vi "Read Map Attributes.vi"(8 "error in":errorcluster, 11 "Tree Map In (empty)":T3) -> (0 "error out":errorcluster, 1 "Modules Types Out":T1[](array[typedef]), 2 "Library References":refnum<vi>[](array[refnum]), 3 "References":T2, 4 "Dependencies?":bool[](array[boolean]), 6 "Descriptions":string[](array[string]))   [LabVIEW 2019, in "Panther Dashboard.lvlib"]
uses:
  Panther Dashboard.lvlib
  <vilib>/National Instruments/Tree Map/Tree Map Data.ctl
  Project References--cluster.ctl
  Module type--enum.ctl
  Map Attribute--enum.ctl
  Panther Dashboard--global.vi
  <vilib>/National Instruments/Tree Map/Tree Map.lvlib
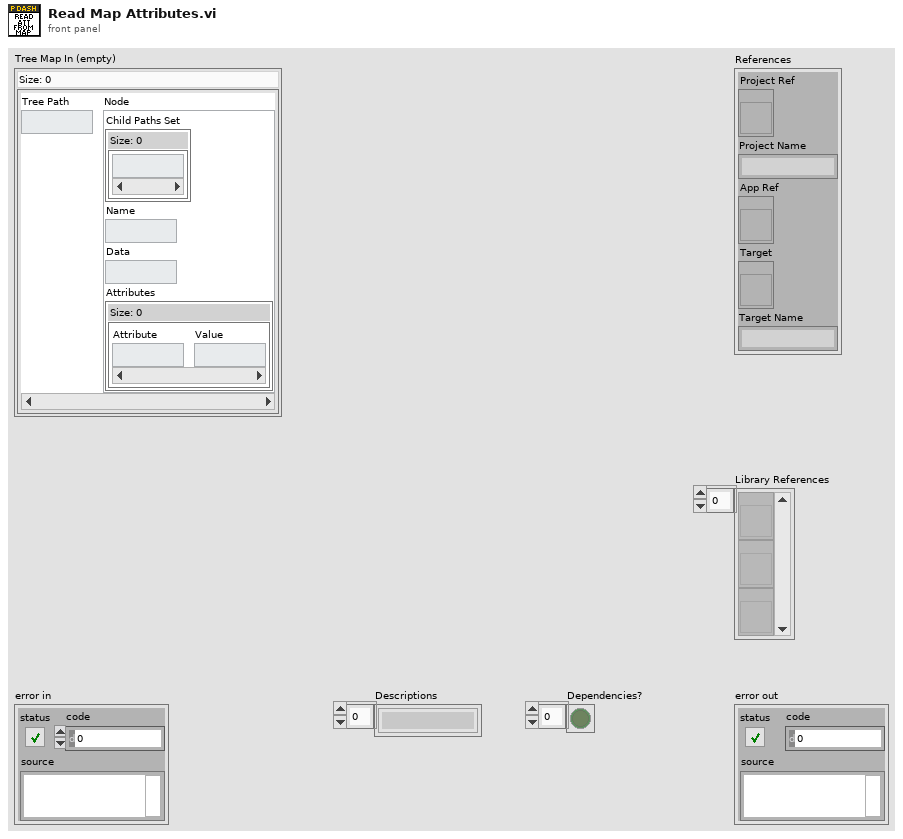
[diagram p1: front panel]
types:
  T1 = typedef "Panther Dashboard.lvlib/Module type--enum.ctl" = enum16{"Singleton", "Cloneable"}
  T2 = typedef "Panther Dashboard.lvlib/Project References--cluster.ctl" = cluster{"Project Ref":refnum<vi>, "Project Name":string, "App Ref":refnum<vi>, "Target":refnum<vi>, "Target Name":string}
  T3 = typedef "Tree Map.lvlib/Tree Map Data.ctl" = map{string, cluster{"Child Paths Set":set{string}, "Name":string, "Data":string, "Attributes":map{string, string}}}
  T4 = typedef "Panther Dashboard.lvlib/Map Attribute--enum.ctl" = enum16{"Path", "ModuleType", "Module Description", "Dependency?", "Target"}
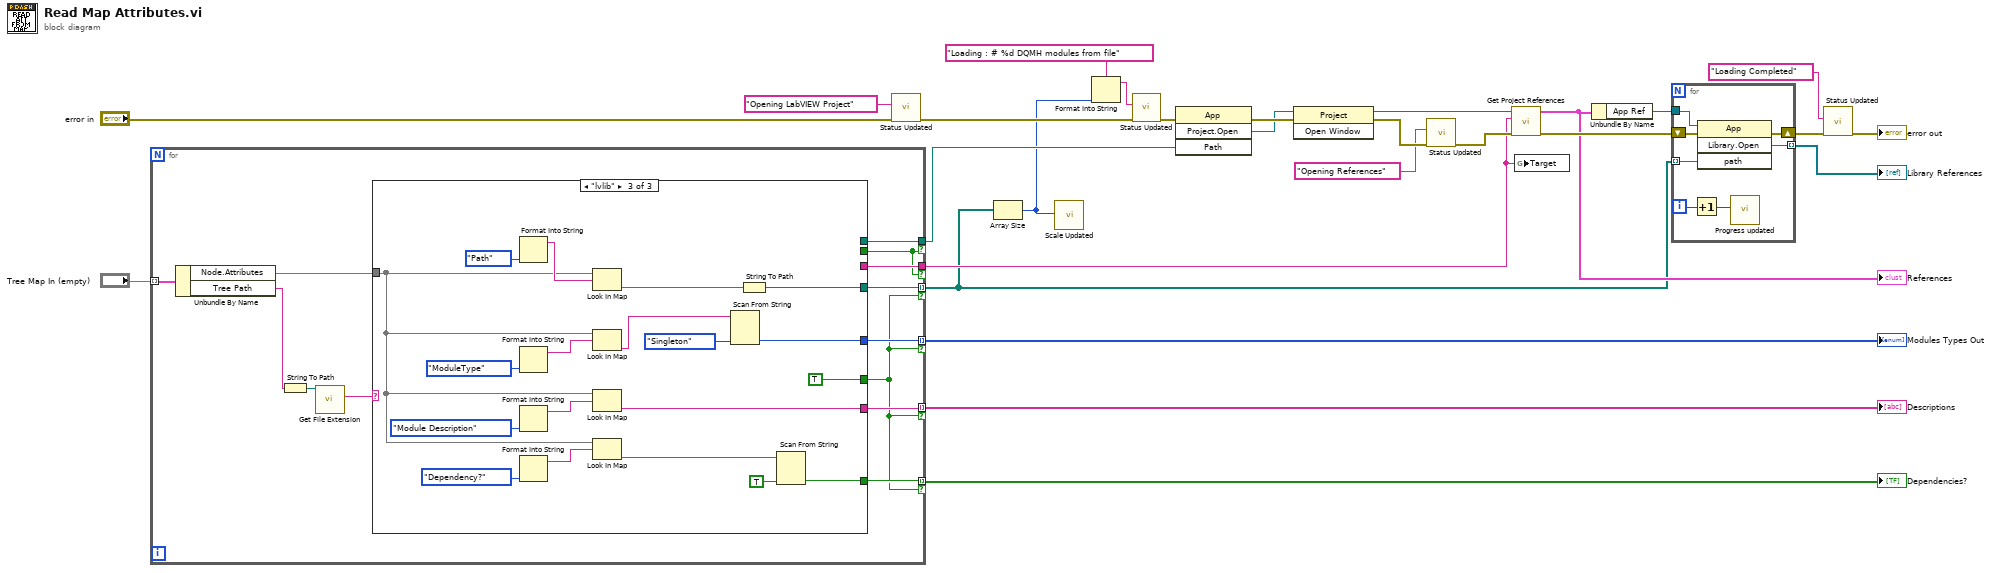
[diagram p0: block diagram]
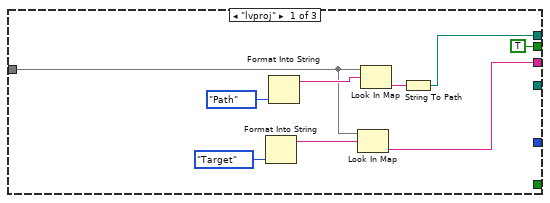
[diagram p2: hidden frame]
diagram:
  n1 = for {
    tunnel: "Tree Map In (empty)" -> [w40] mode=indexing
    tunnel: [w38] -> w16 if=w31
    tunnel: [w37] -> w3 mode=indexing if=w33
    tunnel: [w36] -> w4 mode=indexing if=w33
    tunnel: [w35] -> w15 mode=indexing if=w33
    tunnel: [w34] -> w14 mode=indexing if=w33
    tunnel: [w32] -> w10 if=w31
    n2 = Unbundle By Name(w40) -> ("Node.Attributes"=w39:map{string, string}, "Tree Path"=w29:string)
    n3 = String To Path(string=w29) -> (path=w30:path)
    n4 = call <vilib>:"Get File Extension.vi"("file"=w30) -> ("lowercase file extension"=w28:string)  [unwired: 6 in, 4 out]
    n5 = case shown="\"lvlib\"" w28 {
      tunnel: w39 -> [w42 _ w56]
      tunnel: [w46 _ _] -> w38
      tunnel: [TRUE _ _] -> w31
      tunnel: [_ _ w65] -> w37
      tunnel: [_ _ TRUE] -> w33
      tunnel: [_ _ w62] -> w36
      tunnel: [_ _ w58] -> w35
      tunnel: [_ _ w52] -> w34
      tunnel: [w41 _ _] -> w32
      frame "lvproj" {
        n6 = Format Into String(Map_Attribute--enum."Target" ("Map Attribute")) -> (resulting string=w44:string)  [unwired: 3 in, 1 out]
        n7 = Format Into String(Map_Attribute--enum."Path" ("Map Attribute")) -> (resulting string=w48:string)  [unwired: 3 in, 1 out]
        n8 = Look In Map(map=w42, key=w44) -> (value=w41:string)  [unwired: 1 in, 1 out]
        n9 = Look In Map(map=w42, key=w48) -> (value=w47:string)  [unwired: 1 in, 1 out]
        n10 = String To Path(string=w47) -> (path=w46:path)
      }
      frame Default {
      }
      frame "lvlib" {
        n11 = Format Into String(Map_Attribute--enum."Path" ("Map Attribute")) -> (resulting string=w67:string)  [unwired: 3 in, 1 out]
        n12 = Format Into String(Map_Attribute--enum."ModuleType" ("Map Attribute")) -> (resulting string=w64:string)  [unwired: 3 in, 1 out]
        n13 = Format Into String(Map_Attribute--enum."Module Description" ("Map Attribute")) -> (resulting string=w59:string)  [unwired: 3 in, 1 out]
        n14 = Format Into String(Map_Attribute--enum."Dependency?" ("Map Attribute")) -> (resulting string=w57:string)  [unwired: 3 in, 1 out]
        n15 = Look In Map(map=w56, key=w67) -> (value=w66:string)  [unwired: 1 in, 1 out]
        n16 = Look In Map(map=w56, key=w64) -> (value=w63:string)  [unwired: 1 in, 1 out]
        n17 = Look In Map(map=w56, key=w59) -> (value=w58:string)  [unwired: 1 in, 1 out]
        n18 = Look In Map(map=w56, key=w57) -> (value=w54:string)  [unwired: 1 in, 1 out]
        n19 = Scan From String(input string=w63, default 1=Module_type--enum."Singleton" ("Modules Types Out")) -> (output 1=w62:T1)  [unwired: 3 in, 3 out]
        n20 = String To Path(string=w66) -> (path=w65:path)
        n21 = Scan From String(input string=w54, default 1=TRUE) -> (output 1=w52:bool)  [unwired: 3 in, 3 out]
      }
    }
  }
  "Modules Types Out" <- w4
  "Descriptions" <- w15
  "Dependencies?" <- w14
  n22 = call "Status Updated.vi"("error in (no error)"="error in", "Status"="Opening LabVIEW Project") -> ("error out"=w21:errorcluster)  [unwired: 9 in]
  n23 = Array Size(array=w3) -> (size(s)=w5:i32)
  n24 = call "Scale Updated.vi"("Scale Max"=w5) -> ()  [unwired: 10 in, 1 out]
  n25 = Format Into String(format string="Loading : # %d DQMH modules from file", w5) -> (resulting string=w7:string)  [unwired: 2 in, 1 out]
  n26 = call "Status Updated.vi"("error in (no error)"=w21, "Status"=w7) -> ("error out"=w20:errorcluster)  [unwired: 9 in]
  n27 = invoke class="App" method="Project.Open"(error in=w20, "Path"=w16) -> (error out=w26:errorcluster, "Project:Open"=w11:refnum<vi>)  [unwired: 2 in, 2 out]
  n28 = invoke class="Project" method="Open Window"(reference=w11, error in=w26) -> (reference out=w12:refnum<vi>, error out=w24:errorcluster)  [unwired: 1 in, 1 out]
  n29 = call "Status Updated.vi"("error in (no error)"=w24, "Status"="Opening References") -> ("error out"=w22:errorcluster)  [unwired: 9 in]
  n30 = call "Get Project References.vi"("error in"=w22, "Target Selection"=w10, "Project in"=w12) -> ("error out"=w25:errorcluster, "References"=w13:T2)  [unwired: 7 in]
  "References" <- w13
  n31 = global write "Panther Dashboard--global.vi" "Target"(w10) -> ()
  n32 = Unbundle By Name(w13) -> ("App Ref"=w17:refnum<vi>)
  n33 = for {
    shift-right: [w74] -> w27
    shift-left: w25 -> [w75]
    tunnel: w3 -> [w73] mode=indexing
    tunnel: [w72] -> w18 mode=indexing
    tunnel: w17 -> [w71]
    i -> [w70]
    n34 = Increment(x=w70) -> (x+1=w69:i32)
    n35 = invoke class="App" method="Library.Open"(reference=w71, error in=w75, "path"=w73) -> (error out=w74:errorcluster, "Open Library"=w72:refnum<vi>)  [unwired: 1 in, 2 out]
    n36 = call "Progress updated.vi"("Progress"=w69) -> ()  [unwired: 10 in, 1 out]
  }
  "Library References" <- w18
  n37 = call "Status Updated.vi"("error in (no error)"=w27, "Status"="Loading Completed") -> ("error out"=→"error out":errorcluster)  [unwired: 9 in]
